vi "setRxFIFO.vi"(10 "ReadU16FIFO":refnum<class "IReadU16FIFO.lvclass">, 11 "Modbus in":refnum<class "Modbus.lvclass">) -> (3 "Modbus out":refnum<class "Modbus.lvclass">)   [LabVIEW 2016, in "RTModbus.lvlib" / "Modbus.lvclass"]
uses:
  Modbus.lvclass
  Common_RT_FPGA/IReadU16FIFO/IReadU16FIFO.lvclass
  Modbus.lvclass/Modbus.ctl
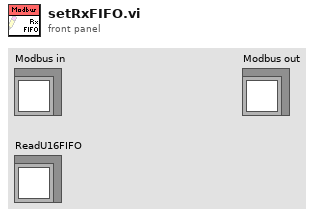
[diagram p1: front panel]
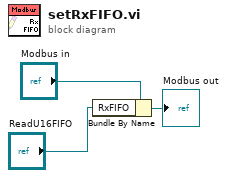
[diagram p0: block diagram]
diagram:
  n1 = Bundle By Name(cluster="Modbus in", "RxFIFO"="ReadU16FIFO") -> (→"Modbus out":refnum<class "Modbus.lvclass">)
